vi "Errors.vi"(0 "Instrument Handle In":i32, 3 "error in":errorcluster) -> (7 "Instrument Handle Out":i32, 8 "Number of Errors":i32, 9 "Errors":i32[](array[numeric]), 10 "error out":errorcluster)   [LabVIEW 8.6, in "ZTScopeM.lvlib"]
doc: "Query all queued errors and clear the error queue."
uses:
  ZTScopeM.lvlib
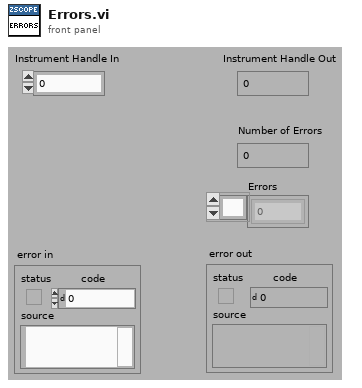
[diagram p1: front panel]
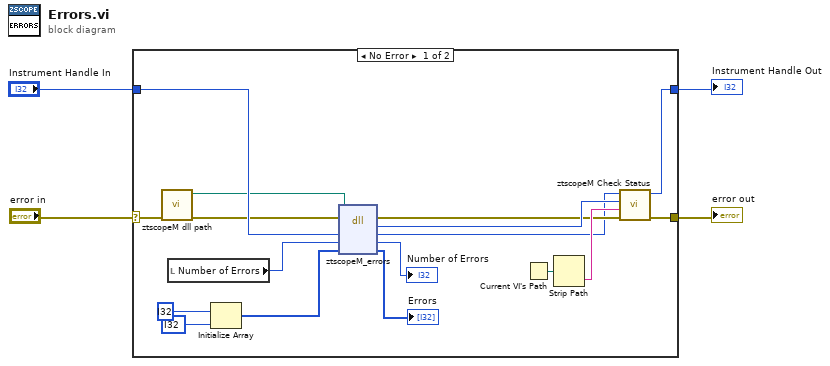
[diagram p0: block diagram]
diagram:
  n1 = case shown="No Error" "error in" {
    selector: "error in" -> [w8 w23]
    tunnel: [w10 w23] -> w1
    tunnel: "Instrument Handle In" -> [w21 w22]
    tunnel: [w5 w22] -> w3
    frame #0 {
      n2 = call "ztscopeM dll path.vi"("error in (no error)"=w8) -> ("error out"=w9:errorcluster, "<instrument>.dll path"=w14:path)  [unwired: 9 in]
      n3 = local read "Number of Errors"() -> (w18:i32)
      n4 = Initialize Array(i32 ?, i32 ? ("dimension size")) -> (w16:i32[])
      n5 = dll-call lib="C:/Program Files (x86)/National Instruments/LabVIEW 2013/instr.lib/ztscopem/ztscopeM.dll" fn="ztscopeM_errors"(path in=w14, error in=w9, "instrumentHandle"=w21, "number_ofErrors"=w18, "errors"=w16) -> (error out=w7:errorcluster, w11:i32, "instrumentHandle"=w6:i32, "number_ofErrors"=→"Number of Errors":i32, "errors"=→"Errors":i32[])  [unwired: 1 in, 1 out]
      n6 = Current VI's Path() -> (path=w13:path)
      n7 = Strip Path(path=w13) -> (name=w12:string)  [unwired: 1 out]
      n8 = call "ztscopeM Check Status.vi"("error in"=w7, "name of VI"=w12, "status (return code)"=w11, "instrument handle in"=w6) -> ("error out"=w10:errorcluster, "instrument handle out"=w5:i32)  [unwired: 2 in]
    }
    frame #1 {
    }
  }
  "Instrument Handle Out" <- w3
  "error out" <- w1
